vi "Initialize.vi"(8 "error in":errorcluster, 11 "Element in":refnum<class "Element.lvclass">) -> (0 "error out":errorcluster, 3 "Element out":refnum<class "Element.lvclass">)   [LabVIEW 2014, in "Element.lvclass"]
uses:
  Element.lvclass
  Controls/Attribute.ctl
  <vilib>/xml/Close Reference(Node).vi
  <vilib>/xml/Close Reference(NNMap).vi
  <resource>/objmgr/DOMUserDefRef.rc
  <vilib>/xml/NI_XML.lvlib
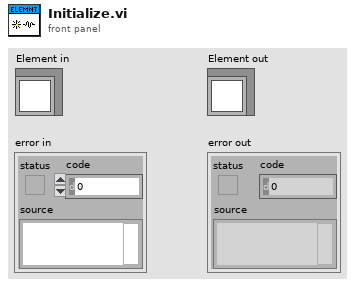
[diagram p1: front panel]
types:
  T1 = typedef "Attribute.ctl" = cluster{"Name":string, "Value":string}
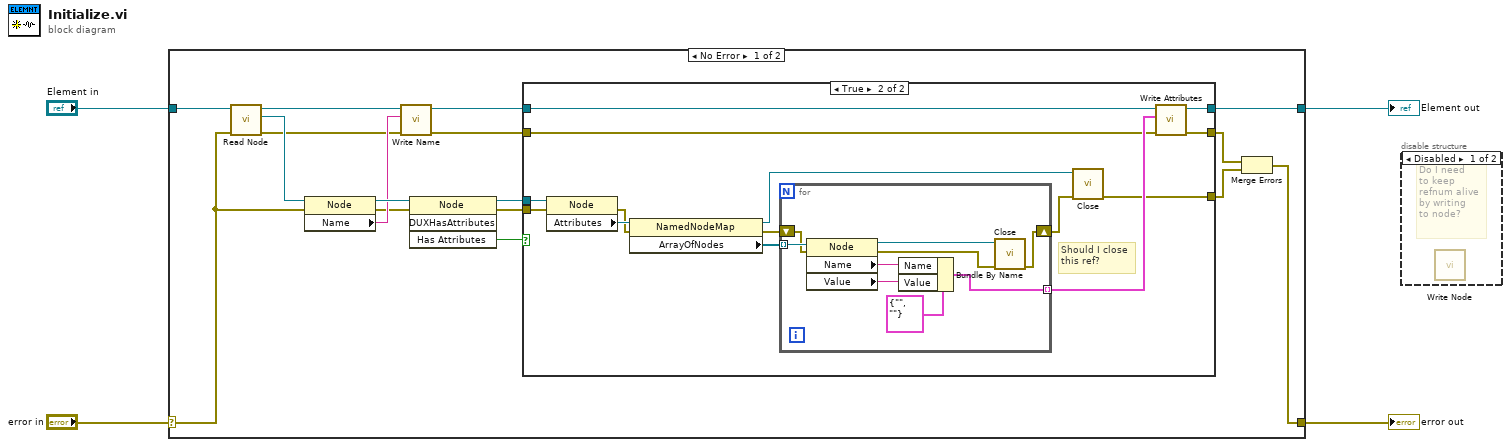
[diagram p0: block diagram]
diagram:
  n1 = case shown="No Error" "error in" {
    selector: "error in" -> [w6 w49]
    tunnel: [w5 w49] -> w3
    tunnel: [w11 w48] -> w1
    tunnel: "Element in" -> [w18 w48]
    frame No Error {
      n2 = call-dynamic "Read Node.vi"("error in"=w6, "Element in"=w18) -> ("error out"=w10:errorcluster, "Node"=w17:refnum<k20>, "Element out"=w16:refnum<class "Element.lvclass">)  [unwired: 7 in]
      n3 = property class="Node"(reference=w17, error in=w6) -> (reference out=w21:refnum<k20>, error out=w12:errorcluster, "Name"=w15:string)
      n4 = call-dynamic "Write Name.vi"("error in"=w10, "Name"=w15, "Element in"=w16) -> ("error out"=w9:errorcluster, "Element out"=w13:refnum<class "Element.lvclass">)  [unwired: 7 in]
      n5 = invoke class="Node" method="DUXHasAttributes"(reference=w21, error in=w12) -> (reference out=w19:refnum<k20>, error out=w14:errorcluster, "Has Attributes"=w20:bool)  [unwired: 2 in, 1 out]
      n6 = case shown="True" w20 {
        tunnel: w19 -> [_ w38]
        tunnel: w14 -> [w22 w35]
        tunnel: w13 -> [w24 w30]
        tunnel: [w24 w28] -> w11
        tunnel: w9 -> [w23 w27]
        tunnel: [w23 w26] -> w8
        tunnel: [w22 w25] -> w7
        frame False {
        }
        frame True {
          # "Should I close\nthis ref?"
          n7 = property class="Node"(reference=w38, error in=w35) -> (error out=w31:errorcluster, "Attributes"=w37:refnum<k20>)  [unwired: 1 out]
          n8 = property class="NamedNodeMap"(reference=w37, error in=w31) -> (reference out=w32:refnum<k20>, error out=w34:errorcluster, "ArrayOfNodes"=w36:refnum<k20>[])
          n9 = for {
            tunnel: w36 -> [w47] mode=indexing
            tunnel: [w42] -> w29 mode=indexing
            shift-right: [w39] -> w33
            shift-left: w34 -> [w40]
            n10 = property class="Node"(reference=w47, error in=w40) -> (reference out=w43:refnum<k20>, error out=w41:errorcluster, "Name"=w45:string, "Value"=w44:string)
            n11 = Bundle By Name(cluster=T1 {"Name"="", "Value"=""} ("Attribute"), "Name"=w45, "Value"=w44) -> (w42:T1)
            n12 = call-poly <vilib>:"Close.vi"("error in (no error)"=w41, "node"=w43) -> ("error out"=w39:errorcluster)  [unwired: 7 in]
          }
          n13 = call-poly <vilib>:"Close.vi"("error in (no error)"=w33, "named node map"=w32) -> ("error out"=w25:errorcluster)  [unwired: 7 in]
          n14 = call-dynamic "Write Attributes.vi"("error in"=w27, "Attributes"=w29, "Element in"=w30) -> ("error out"=w26:errorcluster, "Element out"=w28:refnum<class "Element.lvclass">)  [unwired: 7 in]
        }
      }
      n15 = Merge Errors(w8, w7) -> (w5:errorcluster)
    }
    frame Error {
    }
  }
  "error out" <- w3
  "Element out" <- w1
  n16 = disable-structure shown="Disabled" {
    frame Disabled {
      # "Do I need\nto keep\nrefnum alive\nby writing\nto node?"
      n17 = call-dynamic "Write Node.vi"() -> ()  [unwired: 10 in, 2 out]
    }
    frame Enabled {
    }
  }
